vi "get data.vi"() -> ()   [LabVIEW 2018]
panel:
  out "输出数组":u16[](array[numeric]) format="%04x"
  out "时间":dbl format="%.6f秒"
  in  "点数":i16=10 min=1 max=960 step=1
  in  "软元件":string="D0"
  in  "本地端口":u16=65502
  in  "目的端口":u16=65502
  in  "目的IP地址":string="192.168.3.250"
  out "数据输出":string
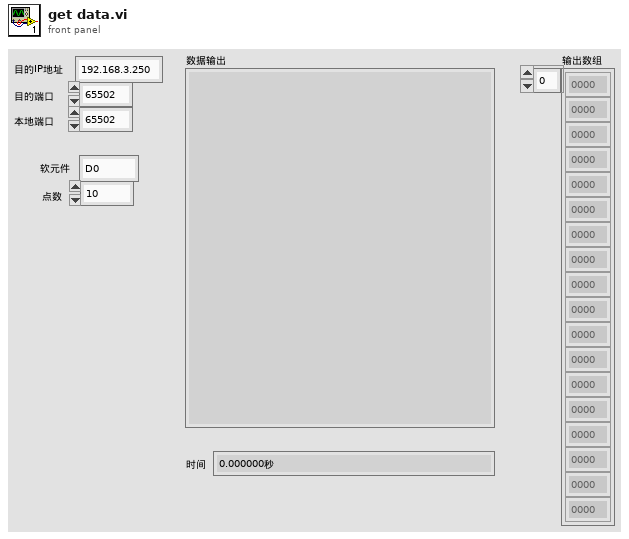
[diagram p1: front panel]
types:
  T1 = cluster{"目的端口":u16, "网络地址":u32, "连接ID":refnum<k16>}
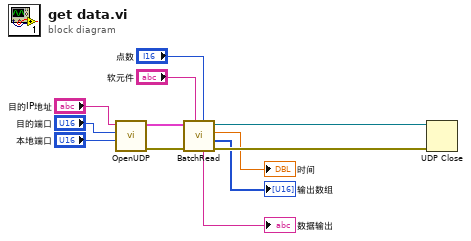
[diagram p0: block diagram]
diagram:
  n1 = call "OpenUDP.vi"("本地端口"="本地端口", "目的端口"="目的端口", "目的IP地址"="目的IP地址") -> ("错误输出"=w12:errorcluster, "连接输出"=w1:T1)  [unwired: 7 in]
  n2 = call "BatchRead.vi"("点数"="点数", "软元件"="软元件", "错误输入"=w12, "连接"=w1) -> ("错误输出"=w10:errorcluster, "输出数组"=→"输出数组":u16[], "时间"=→"时间":dbl, "连接ID 2"=w11:refnum<k16>, "数据输出"=→"数据输出":string)  [unwired: 3 in]
  n3 = UDP Close(connection ID=w11, 8:w10) -> ()  [unwired: 2 out]
